vi "GasteilerStringSpeichern.vi"(10 "Abschnitt":string, 11 "GasteilerDefinition":string[][](array[string])) -> (3 "Gasdivider Text to save":string[](array[string]))   [LabVIEW 2020, in "System Einstellungen V2.lvlib"]
uses:
  System Einstellungen V2.lvlib
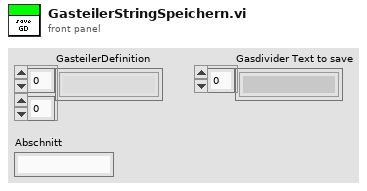
[diagram p1: front panel]
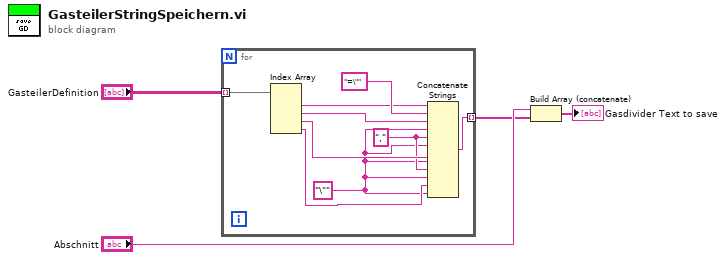
[diagram p0: block diagram]
diagram:
  n1 = for {
    tunnel: "GasteilerDefinition" -> [w12] mode=indexing
    tunnel: [w9] -> w2 mode=indexing
    w7 = "," ("String")
    w5 = "\""
    n2 = Index Array(array=w12) -> (element #1=w11:string, element #2=w10:string, element #3=w8:string, element #4=w6:string)  [unwired: 4 in]
    n3 = Concatenate Strings(w11, "=\"", w10, w5, w7, w5, w8, w5, w7, w5, w6, w5) -> (w9:string)
  }
  n4 = Build Array (concatenate)("Abschnitt", w2) -> (→"Gasdivider Text to save":string[])
